vi "TLB Native Dynamic Events ver 0.05f.vi"() -> ()   [LabVIEW 2018]
uses:
  Labview Training Phase 2/Enum Controls/States for Action Engine.ctl
  Type def/TLB event states.ctl
  Type def/TLB MHL States.ctl
  <vilib>/Studica/Studica Toolkit/Background/I2C Channel.ctl
  <vilib>/Studica/Studica Toolkit/NavX/NavX.lvlib
  <vilib>/myRIO/Common/Instrument Driver Framework/myRIO v1.0/AI/typedefs/AI Channels Enum.ctl
  <vilib>/myRIO/Common/Instrument Driver Framework/myRIO v1.0/AI/typedefs/AI Channels List.ctl
  <vilib>/Studica/Studica Toolkit/Background/Mxp Selection.ctl
  <vilib>/ptbypt/NI_PtbyPt.lvlib
  Type def/Type def.ctl
  Type def/Motor Control Cluster.ctl
  <vilib>/Studica/Studica Blackhawk/Blackhawk.lvlib
  <vilib>/Studica/Studica Toolkit/Background/DIO Channel.ctl
panel:
  out "Image Processing error":errorcluster
  in  "Camera playback":bool
  out "Image Out":T1(plugin-control)
  out "element":T2
  in  "Servo Angle":u8(slide) scale=0.0..180.0
  in  "On/Off":bool
  out "Blackhawk error":errorcluster
  out "Value Read":bool
  out "Object detected":bool
  out "Yaw":dbl
  in  "NavX Zero Yaw":bool
  out "NavX Info Out":T4
  out "LinearAcceleration":T5
  out "Displacement":T6
  out "YRPHfH":T7
  out "Distance":T8
  in  "Return to IDLE":bool
  out "Right IR Sensor":dbl
  out "Left IR Sensor":dbl
  out "CM":fxp<+,64,16>
  out "Ultrasonic sensor":dbl format="%0.2f"
  in  "xTargetSpeed":dbl
  in  "yTargetSpeed":dbl
  in  "wTargetSpeed":dbl
  out "Speed":T9
  in  "Reset Encoder 0":bool
  out "Action Queue Items":i32
  out "State Logic Queue Items":i32
  out "Action Queues items":string[](array[string])=["Hardware reset", "Software reset", ""]
  out "State logic":T10=enum."Task 2"
  out "Action State":string
  in  "Tasks Selector":string(combo)="Task 2"
  in  "Stop Queue":bool
  in  "Start Task":bool
  # "Test Programme written by Calvin Loke    Dated: 28 Aug 2019\nTest Programme revised by Dr Alex See   Dated 30 Aug 2019\n\nProgramme version:   TLB Native Dynamic Events ver 0.04b.vi"
  # "Sequence of Actions"
  # "Continuous (Repeated)"
  # "System Health Status Update"
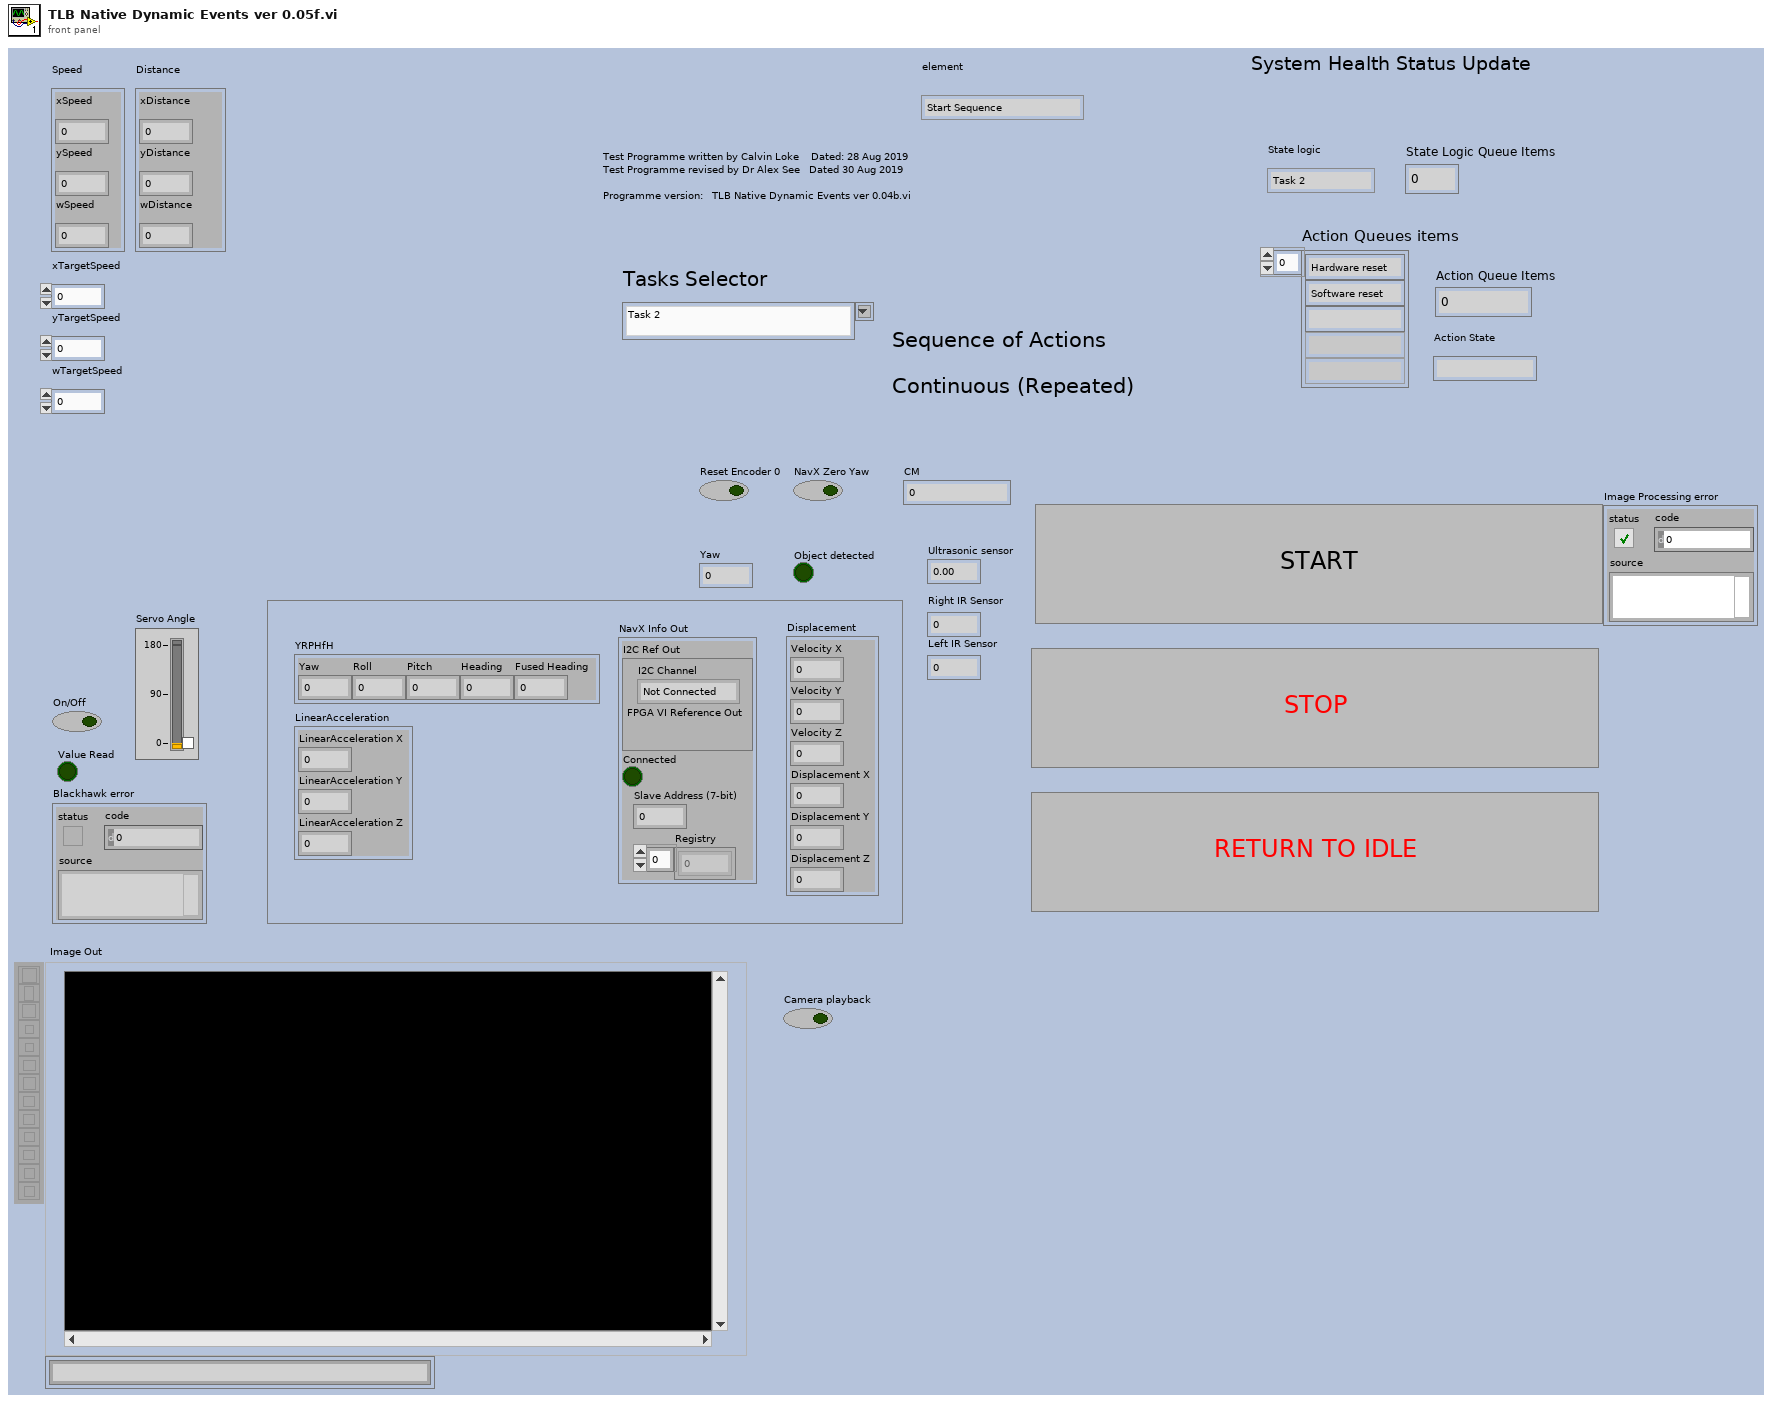
[diagram p1: front panel]
types:
  T1 = typedef "IMAQ Image.ctl" = refnum<image>
  T2 = typedef "TLB event states.ctl" = enum16{"Start Sequence", "Exit", "Start Task 1", "Start Task 2", "Start Task 3", "Start Task 4", "Camera vision", "Wall follow mode", "Idle", "Start Drive Straight"}
  T3 = typedef "I2C Channel.ctl" = enum16{"Not Connected", "A", "B"}
  T4 = cluster{"I2C Ref Out":cluster{"I2C Channel":T3, "FPGA VI Reference Out":refnum<k20>}, "Connected":bool, "Slave Address (7-bit)":u8, "Registry":u8[]}
  T5 = cluster{"LinearAcceleration X":dbl, "LinearAcceleration Y":dbl, "LinearAcceleration Z":dbl}
  T6 = cluster{"Velocity X":dbl, "Velocity Y":dbl, "Velocity Z":dbl, "Displacement X":dbl, "Displacement Y":dbl, "Displacement Z":dbl}
  T7 = cluster{"Yaw":dbl, "Roll":dbl, "Pitch":dbl, "Heading":dbl, "Fused Heading":dbl}
  T8 = cluster{"xDistance":dbl, "yDistance":dbl, "wDistance":dbl}
  T9 = cluster{"xSpeed":dbl, "ySpeed":dbl, "wSpeed":dbl}
  T10 = typedef "TLB MHL States.ctl" = enum16{"None", "Startup", "Idle", "Processing", "Shutdown", "Reset", "Task 1", "Task 2", "Task 3", "Task 4", "Task 4a", "Task 4b", "Task 4c", "Task 4d", "Task 4e", "Task 4f", "Task 4g", "Task 4h", "Acquire image", "Wall follow mode", "Autodrive", "Autodrive a"}
  T11 = typedef "States for Action Engine.ctl" = enum16{"Initialize", "Write", "Read"}
  T12 = typedef "DIO Channel.ctl" = enum16{"Not Connected", "A/DIO1", "A/DIO2", "A/DIO3", "A/DIO4", "A/DIO5", "A/DIO6", "A/DIO7", "A/DIO13", "B/DIO1", "B/DIO2", "B/DIO3", "B/DIO4", "B/DIO5", "B/DIO6", "B/DIO7", "B/DIO13", "C/DIO0", "C/DIO1", "C/DIO2", "C/DIO3", "C/DIO4", "C/DIO5", "C/DIO6", "C/DIO7"}
  T13 = typedef "Motor Control Cluster.ctl" = cluster{"Vx":dbl, "Vy":dbl, "Vw":dbl}
  T14 = typedef "Type def.ctl" = cluster{"Front Ultrasonic Obstruct":bool, "Left Ultrasonic Obstruct":bool, "Right Ultrasonic Obstruct ":bool}
  T15 = typedef "Mxp Selection.ctl" = enum16{"MXP A", "MXP B"}
  T16 = typedef "TLB event states.ctl" = enum16{"Start Sequence", "Exit", "Start Task 1", "Start Task 2", "Start Task 3", "Start Task 4", "RT Camera tracking", "Wall follow mode", "Idle"}
  T17 = cluster{"I2C Channel":T3, "FPGA VI Reference Out":refnum<k20>}
  T18 = typedef "AI Channels List.ctl" = T19[]
  T19 = typedef "AI Channels Enum.ctl" = enum16{"Not Connected", "AudioIn/Left", "AudioIn/Right", "C/AI0", "C/AI1", "A/AI0", "A/AI1", "A/AI2", "A/AI3", "A/AI4", "A/AI5", "A/AI6", "A/AI7", "B/AI0", "B/AI1", "B/AI2", "B/AI3", "B/AI4", "B/AI5", "B/AI6", "B/AI7", "AI/AI0", "AI/AI1", "AI/AI2", "AI/AI3", "A/AI0 (DIFF)", "A/AI1 (DIFF)", "A/AI2 (DIFF)", "A/AI3 (DIFF)", "B/AI0 (DIFF)", "B/AI1 (DIFF)", "B/AI2 (DIFF)", "B/AI3 (DIFF)"}
  T20 = cluster{"DIO Channel":T12, "FPGA VI Reference Out":refnum<k20>}
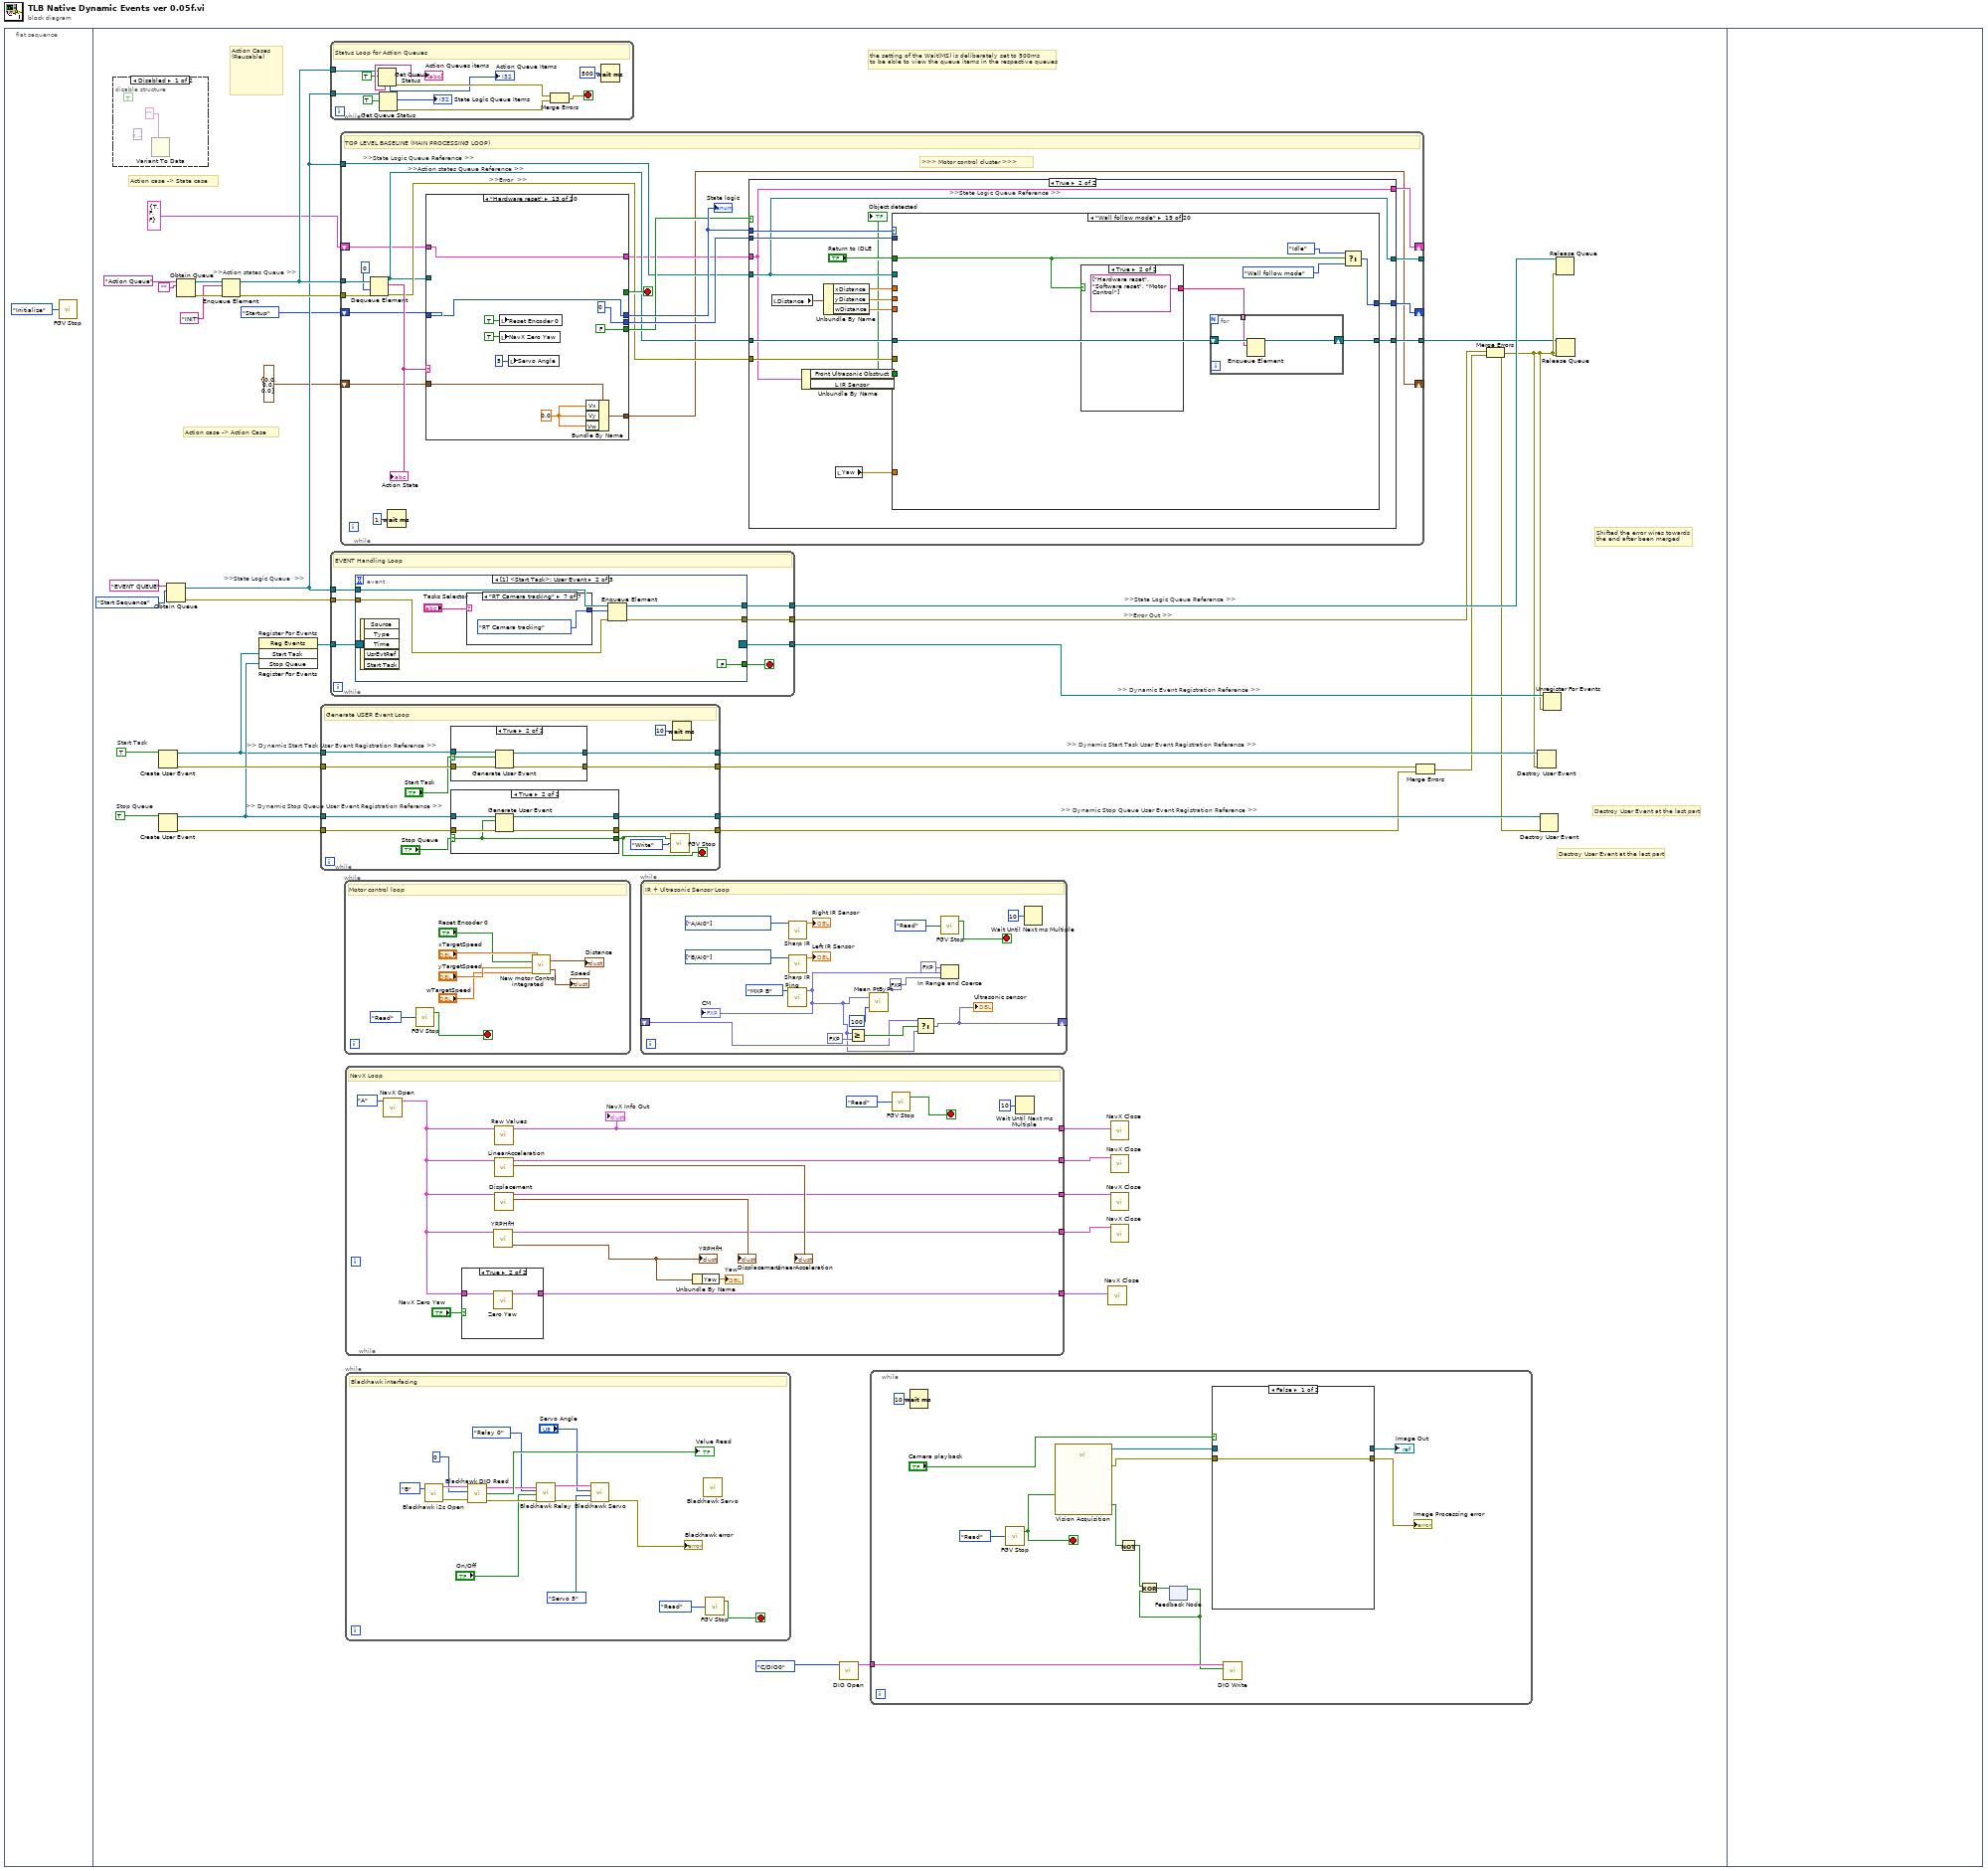
[diagram p0: block diagram]
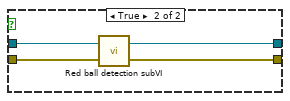
[diagram p2: hidden frame]
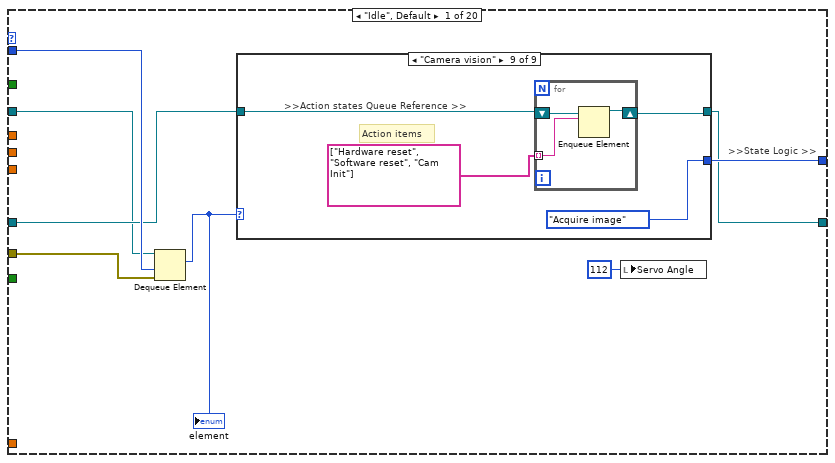
[diagram p6: hidden frame]
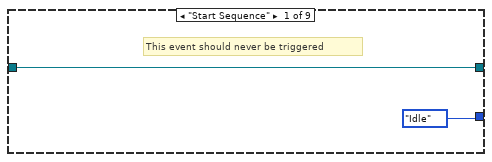
[diagram p7: hidden frame]
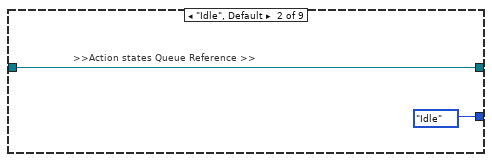
[diagram p8: hidden frame]
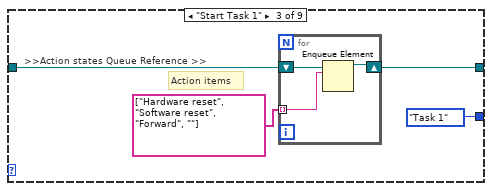
[diagram p9: hidden frame]
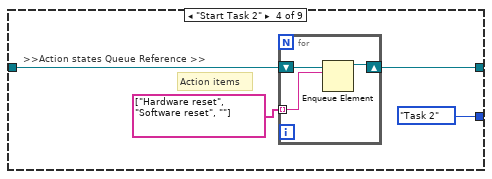
[diagram p10: hidden frame]
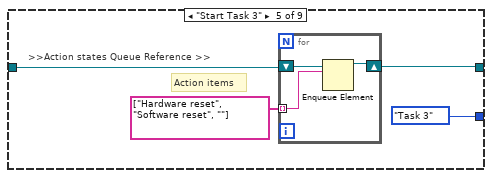
[diagram p11: hidden frame]
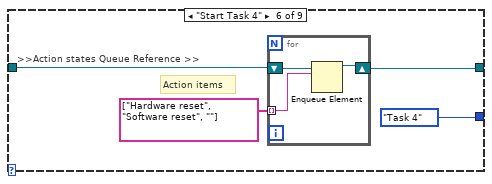
[diagram p12: hidden frame]
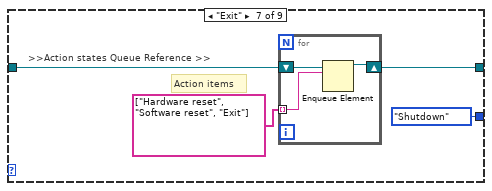
[diagram p13: hidden frame]
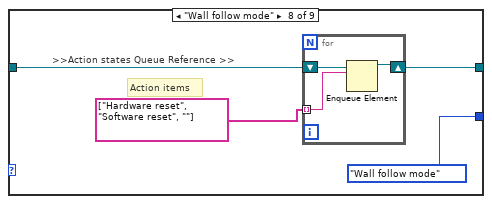
[diagram p14: hidden frame]
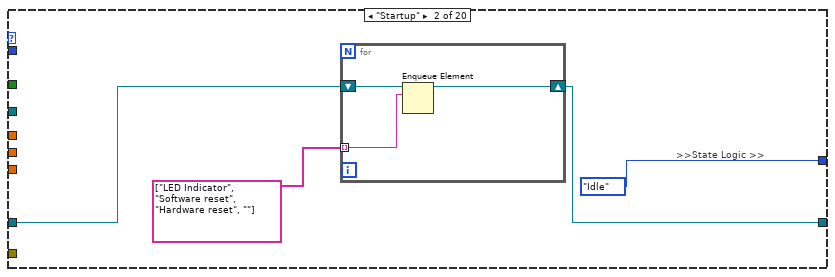
[diagram p15: hidden frame]
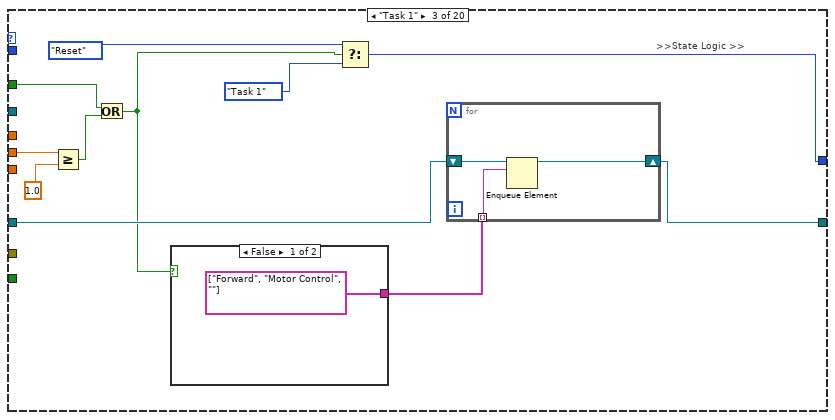
[diagram p16: hidden frame]
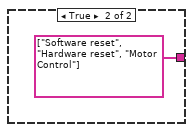
[diagram p17: hidden frame]
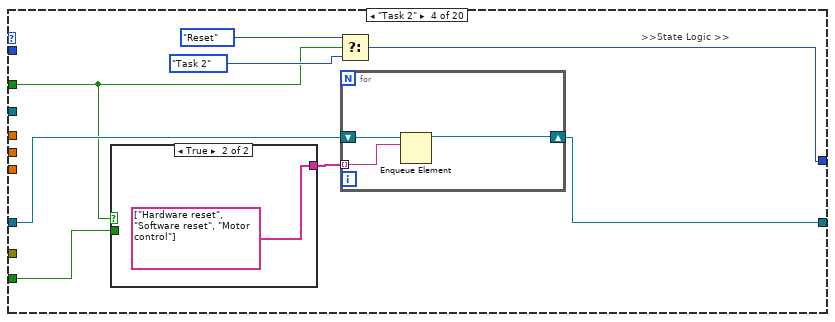
[diagram p18: hidden frame]
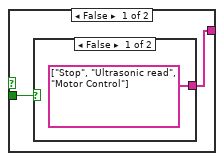
[diagram p19: hidden frame]
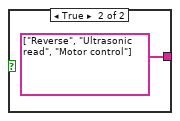
[diagram p20: hidden frame]
diagram:
  n1 = flat-sequence {
    frame #0 {
      n2 = call "FGV Stop.vi"("Init/Read/Write State"=States_for_Action_Engine."Initialize") -> ()  [unwired: 2 in, 2 out]
    }
    frame #1 {
      w39 = TRUE  # Stop Queue
      w38 = TRUE  # Start Task
      # "Action case -> Action Case"
      # "Action case -> State case"
      # "the setting of the Wait(MS) is deliberately set to 500ms\nto be able to view the queue items in the respective queues"
      # "Action Cases\n(Reusable)"
      # ">>Error Out >>"
      # ">> Dynamic Stop Queue User Event Registration Reference >>"
      # ">> Dynamic Start Task User Event Registration Reference >>"
      # ">> Dynamic Stop Queue User Event Registration Reference >>"
      # ">> Dynamic Start Task User Event Registration Reference >>"
      # ">> Dynamic Event Registration Reference >>"
      # ">>Action states Queue >>"
      # ">>State Logic Queue  >>"
      # ">>State Logic Queue Reference >>"
      # "Destroy User Event at the last part"
      # "Destroy User Event at the last part"
      # "Shifted the error wires towards\nthe end after been merged"
      n3 = disable-structure shown="Disabled" {
        frame Disabled {
          (unwired) variant
          (unwired) TRUE
          n4 = Variant To Data(type="") -> ()  [unwired: 2 in, 2 out]
        }
        frame Enabled {
        }
      }
      n5 = Create User Event(user event datatype=w38) -> (user event=w30:refnum<user-event>, error out=w35:errorcluster)  [unwired: 1 in]
      n6 = Create User Event(user event datatype=w39) -> (user event=w31:refnum<user-event>, error out=w34:errorcluster)  [unwired: 1 in]
      n7 = Obtain Queue(name (unnamed)="EVENT QUEUE", element data type=TLB_event_states."Start Sequence" ("Enum")) -> (queue out=w15:refnum<queue>, error out=w21:errorcluster)  [unwired: 3 in, 1 out]
      n8 = Obtain Queue(name (unnamed)="Action Queue", element data type="") -> (queue out=w24:refnum<queue>, error out=w20:errorcluster)  [unwired: 3 in, 1 out]
      n9 = Enqueue Element(queue=w24, element="INIT", error in (no error)=w20) -> (queue out=w16:refnum<queue>, error out=w19:errorcluster)  [unwired: 1 in, 1 out]
      n10 = register-events "Register For Events"(w30, w31) -> (reference out=w29:refnum<event-registration>)  [unwired: 2 in, 1 out]
      n11 = while {
        tunnel: w30 -> [w603]
        tunnel: w31 -> [w602]
        tunnel: [w601] -> w37
        tunnel: [w600] -> w36
        tunnel: w35 -> [w599]
        tunnel: [w598] -> w33
        tunnel: w34 -> [w597]
        tunnel: [w596] -> w32
        stop <- w592 stop-if-true
        # "Generate USER Event Loop"
        n12 = case shown="True" "Start Task" {
          selector: "Start Task" -> [_ w615]
          tunnel: w603 -> [w614 w619]
          tunnel: [w614 w618] -> w600
          tunnel: w599 -> [w613 w617]
          tunnel: [w613 w616] -> w598
          frame False {
          }
          frame True {
            n13 = Generate User Event(user event=w619, event data cluster=w615, error in=w617) -> (user event out=w618:refnum<user-event>, error out=w616:errorcluster)  [unwired: 1 in]
          }
        }
        n14 = case shown="True" "Stop Queue" {
          selector: "Stop Queue" -> [_ w608]
          tunnel: w602 -> [w607 w612]
          tunnel: [w607 w611] -> w601
          tunnel: w597 -> [w606 w610]
          tunnel: [w606 w609] -> w596
          tunnel: [FALSE w608] -> w592
          frame False {
          }
          frame True {
            n15 = Generate User Event(user event=w612, event data cluster=w608, error in=w610) -> (user event out=w611:refnum<user-event>, error out=w609:errorcluster)  [unwired: 1 in]
          }
        }
        n16 = call "FGV Stop.vi"("Init/Read/Write State"=States_for_Action_Engine."Write", "Input Node"=w592) -> ()  [unwired: 1 in, 2 out]
        n17 = Wait (ms)(milliseconds to wait=u32 10) -> ()  [unwired: 1 out]
      }
      n18 = while {
        tunnel: w16 -> [w125]
        tunnel: w15 -> [w122]
        stop <- w119 stop-if-true
        # "Status Loop for Action Queues"
        n19 = Get Queue Status(queue=w125, return elements? (F)=TRUE) -> (error out=w121:errorcluster, # elements in queue=→"Action Queue Items":i32, elements=→"Action Queues items":string[])  [unwired: 1 in, 5 out]
        n20 = Get Queue Status(queue=w122, return elements? (F)=TRUE) -> (# pending remove=→"State Logic Queue Items":i32, error out=w120:errorcluster)  [unwired: 1 in, 6 out]
        n21 = Merge Errors(w121, w120) -> (w119:errorcluster)
        n22 = Wait (ms)(milliseconds to wait=u32 500) -> ()  [unwired: 1 out]
      }
      n23 = while {
        tunnel: w29 -> [w565]
        tunnel: [w564] -> w28
        tunnel: w15 -> [w562]
        tunnel: [w561] -> w27
        tunnel: w21 -> [w560]
        tunnel: [w559] -> w18
        stop <- w563 stop-if-true
        # "EVENT Handling Loop"
        n24 = event shown="[1] <Start Task>: User Event" {
          selector: w565 -> [_ _ _]
          dyn-events: [_ _ _] -> w564
          timeout: _ -> [_ _ _]
          tunnel: [FALSE FALSE w591] -> w563
          tunnel: w562 -> [w570 w577 w589]
          tunnel: [w569 w576 w590] -> w561
          tunnel: w560 -> [w567 w573 w587]
          tunnel: [w566 w572 w586] -> w559
          event Timeout {
            n25 = event-data() -> ()  [unwired: 1 in, 3 out]
            n26 = Enqueue Element(queue=w570, element=TLB_event_states."Idle" ("Enum"), error in (no error)=w567) -> (queue out=w569:refnum<queue>, error out=w566:errorcluster)  [unwired: 1 in, 1 out]
          }
          event User Event {
            n27 = event-data() -> ()  [unwired: 1 in, 5 out]
            n28 = case shown="\"RT Camera tracking\"" "Tasks Selector" {
              tunnel: [TLB_event_states."Idle" ("Enum") TLB_event_states."Start Task 1" ("Enum") TLB_event_states."Start Task 2" ("Enum") TLB_event_states."Start Task 3" ("Enum") TLB_event_states."Start Task 4" ("Enum") TLB_event_states."Wall follow mode" ("Enum") TLB_event_states."RT Camera tracking" ("Enum")] -> w574
              frame Default {
              }
              frame "Task 1" {
              }
              frame "Task 2" {
              }
              frame "Task 3" {
              }
              frame "Task 4" {
              }
              frame "Wall following" {
              }
              frame "RT Camera tracking" {
              }
            }
            n29 = Enqueue Element(queue=w577, element=w574, error in (no error)=w573) -> (queue out=w576:refnum<queue>, error out=w572:errorcluster)  [unwired: 1 in, 1 out]
          }
          event User Event {
            n30 = event-data() -> ("Stop Queue"=w591:bool)  [unwired: 1 in, 4 out]
            n31 = Enqueue Element At Opposite End(queue=w589, element=TLB_event_states."Exit" ("Enum"), error in (no error)=w587) -> (queue out=w590:refnum<queue>, error out=w586:errorcluster)  [unwired: 1 in, 1 out]
          }
        }
      }
      n32 = while {
        tunnel: w15 -> [w136]
        shift-right: [w141] -> _
        shift-left: TLB_MHL_States."Startup" ("Enum") -> [w133]
        tunnel: w16 -> [w146]
        tunnel: w19 -> [w144]
        tunnel: [w143] -> _
        tunnel: [w142] -> w13
        shift-right: [w130] -> _
        shift-left: T14 {"Front Ultrasonic Obstruct"=TRUE, "Left Ultrasonic Obstruct"=FALSE, "Right Ultrasonic Obstruct "=FALSE} -> [w132]
        shift-right: [w128] -> _
        shift-left: T13 {"Vx"=0.0, "Vy"=0.0, "Vw"=0.0} -> [w129]
        stop <- w139 stop-if-true
        # ">>> Motor control cluster >>>"
        # ">>Error  >>"
        # ">>Action states Queue Reference >>"
        # ">>State Logic Queue Reference >>"
        # "TOP LEVEL BASELINE (MAIN PROCESSING LOOP)"
        n33 = Dequeue Element(queue=w146, timeout in ms (-1)=0, error in (no error)=w144) -> (queue out=w134:refnum<queue>, element=w145:string, error out=w135:errorcluster)  [unwired: 1 out]
        "Action State" <- w145
        n34 = Wait (ms)(milliseconds to wait=u32 1) -> ()  [unwired: 1 out]
        n35 = case shown="\"Hardware reset\"" w145 {
          tunnel: [w405 w412 w417 w425 w434 w444 w453 w460 w471 w479 w487 w496 w506 TLB_MHL_States."Shutdown" ("Enum") w521 w525 w539 w545 w549 w558] -> w147
          tunnel: [w404 0 0 0 0 0 0 0 0 0 0 0 0 0 0 0 0 0 0 0] -> w140
          tunnel: [_ _ _ _ _ _ _ _ _ _ _ _ _ TRUE _ _ _ _ _ _] -> w139
          tunnel: [TRUE FALSE FALSE FALSE FALSE FALSE FALSE FALSE FALSE FALSE FALSE FALSE FALSE FALSE FALSE FALSE FALSE FALSE FALSE FALSE] -> w138
          tunnel: w134 -> [_ _ _ _ _ _ _ _ _ _ _ _ _ _ _ _ _ _ _ _]
          tunnel: w133 -> [w405 w412 w417 w425 w434 w444 w453 w460 w471 w479 w487 w496 w506 _ w521 w525 w539 w545 w549 w558]
          tunnel: w132 -> [w402 w409 w414 w421 w430 w439 w448 w457 w466 w475 w488 w493 w501 w508 w520 w528 w540 w546 w547 w553]
          tunnel: [w402 w409 w414 w421 w430 w439 w448 w457 w466 w475 w488 w492 w501 w508 w517 w527 w540 w546 w547 w553] -> w131
          tunnel: w129 -> [w401 w408 w413 w419 w428 w437 w447 w455 w465 w473 w481 w490 w500 w507 w513 w522 w531 w544 w552 w555]
          tunnel: [w401 w408 w413 w420 w429 w438 w446 w456 w464 w474 w481 w490 w498 w507 w513 w522 w532 w544 w552 w555] -> w128
          frame "No action", Default {
            n36 = case shown="\"Startup\", Default" w405 {
              tunnel: [0 100] -> w404
              frame "Startup", Default {
              }
              frame "Idle" {
              }
            }
          }
          frame "Init" {
            # ">>State Logic  >>"
          }
          frame "LED Indicator" {
          }
          frame "Forward" {
            n37 = local write "Reset Encoder 0"(FALSE ("Reset Encoder 0")) -> ()
            n38 = local write "NavX Zero Yaw"(FALSE ("NavX Zero Yaw")) -> ()
            n39 = Bundle By Name(cluster=w419, "Vy"=0.6) -> (w420:T13)
          }
          frame "Reverse" {
            n40 = local write "NavX Zero Yaw"(FALSE ("NavX Zero Yaw")) -> ()
            n41 = local write "Reset Encoder 0"(FALSE ("Reset Encoder 0")) -> ()
            n42 = Bundle By Name(cluster=w428, "Vy"=-0.6) -> (w429:T13)
          }
          frame "Right" {
            n43 = local write "NavX Zero Yaw"(FALSE ("NavX Zero Yaw")) -> ()
            n44 = local write "Reset Encoder 0"(FALSE ("Reset Encoder 0")) -> ()
            n45 = Bundle By Name(cluster=w437, "Vx"=0.6) -> (w438:T13)
          }
          frame "Left" {
            n46 = Bundle By Name(cluster=w447, "Vx"=-0.6) -> (w446:T13)
            n47 = local write "NavX Zero Yaw"(FALSE ("NavX Zero Yaw")) -> ()
            n48 = local write "Reset Encoder 0"(FALSE ("Reset Encoder 0")) -> ()
          }
          frame "Rotate CW" {
            n49 = local write "NavX Zero Yaw"(FALSE ("NavX Zero Yaw")) -> ()
            n50 = local write "Reset Encoder 0"(FALSE ("Reset Encoder 0")) -> ()
            n51 = Bundle By Name(cluster=w455, "Vw"=-0.3) -> (w456:T13)
          }
          frame "Rotate ACW" {
            n52 = local write "Reset Encoder 0"(FALSE ("Reset Encoder 0")) -> ()
            n53 = local write "NavX Zero Yaw"(FALSE ("NavX Zero Yaw")) -> ()
            n54 = Bundle By Name(cluster=w465, "Vw"=0.15) -> (w464:T13)
          }
          frame "Stop" {
            w472 = 0.0
            n55 = local write "NavX Zero Yaw"(FALSE ("NavX Zero Yaw")) -> ()
            n56 = local write "Reset Encoder 0"(FALSE ("Reset Encoder 0")) -> ()
            n57 = Bundle By Name(cluster=w473, "Vx"=w472, "Vy"=w472, "Vw"=w472) -> (w474:T13)
          }
          frame "Motor control" {
            # "Replace with FGV"
            n58 = Unbundle By Name(w481) -> ("Vx"=w484:dbl, "Vy"=w483:dbl, "Vw"=w482:dbl)
            n59 = local write "xTargetSpeed"(w484) -> ()
            n60 = local write "yTargetSpeed"(w483) -> ()
            n61 = local write "wTargetSpeed"(w482) -> ()
          }
          frame "Software reset" {
            w491 = FALSE ("NavX Zero Yaw")
            n62 = local write "NavX Zero Yaw"(w491) -> ()
            n63 = Bundle By Name(cluster=w493, "Front Ultrasonic Obstruct"=w491, "L IR Sensor"=0.0) -> (w492:T14)
          }
          frame "Hardware reset" {
            w499 = 0.0
            n64 = local write "Reset Encoder 0"(TRUE ("Reset Encoder 0")) -> ()
            n65 = local write "NavX Zero Yaw"(TRUE ("NavX Zero Yaw")) -> ()
            n66 = local write "Servo Angle"(u8 5 ("Servo Angle")) -> ()
            n67 = Bundle By Name(cluster=w500, "Vx"=w499, "Vy"=w499, "Vw"=w499) -> (w498:T13)
          }
          frame "Exit" {
          }
          frame "Ultrasonic read" {
            # "Object detection"
            n68 = local read "Ultrasonic sensor"() -> (w516:dbl)
            n69 = Less Or Equal?(x=w516, y=20.0) -> (x <= y?=w514:bool)
            n70 = Bundle By Name(cluster=w520, "Front Ultrasonic Obstruct"=w514) -> (w517:T14)
          }
          frame "IR Sensor Read" {
            n71 = local read "Left IR Sensor"() -> (w526:dbl)
            n72 = Bundle By Name(cluster=w528, "L IR Sensor"=w526) -> (w527:T14)
          }
          frame "Calculate" {
            n73 = Unbundle By Name(w540) -> ("L IR Sensor"=w536:dbl)
            n74 = Subtract(x=w536, y=20.0) -> (x-y=w534:dbl)
            n75 = Multiply(x=w534, y=0.01) -> (x*y=w530:dbl)
            n76 = Bundle By Name(cluster=w531, "Vy"=0.4, "Vw"=w530) -> (w532:T13)
          }
          frame "Cam Init" {
            n77 = local write "Camera playback"(TRUE ("Camera playback")) -> ()
          }
          frame "Cam Acq" {
            n78 = local write "Camera playback"(TRUE ("Camera playback")) -> ()
          }
          frame "Cam Exit" {
            n79 = local write "Camera playback"(FALSE ("Camera playback")) -> ()
          }
        }
        "State logic" <- w147
        n80 = case shown="True" w138 {
          tunnel: w147 -> [w151 w167]
          tunnel: w136 -> [w152 w161]
          tunnel: w134 -> [w150 w166]
          tunnel: [w152 w161] -> w143
          tunnel: [w150 w165] -> w142
          tunnel: [w151 w164] -> w141
          tunnel: w135 -> [_ w163]
          tunnel: w140 -> [_ w162]
          tunnel: w131 -> [w149 w153]
          tunnel: [w149 w153] -> w130
          frame False {
          }
          frame True {
            # ">>State Logic Queue Reference >>"
            n81 = local read "Distance"() -> (w159:T8)
            n82 = Unbundle By Name(w153) -> ("Front Ultrasonic Obstruct"=w154:bool)  [unwired: 1 out]
            "Object detected" <- w154
            n83 = Unbundle By Name(w159) -> ("xDistance"=w156:dbl, "yDistance"=w158:dbl, "wDistance"=w157:dbl)
            n84 = local read "Yaw"() -> (w155:dbl)
            n85 = case shown="\"Wall follow mode\"" w167 {
              tunnel: w161 -> [w169 _ _ _ _ _ _ _ _ _ _ _ _ _ _ _ _ _ _ _]
              tunnel: w166 -> [w171 w230 w242 w255 w277 w286 w300 w315 w328 w341 w352 w358 w361 w367 w370 w372 w374 w376 w379 w393]
              tunnel: [w170 w229 w241 w256 w276 w287 w299 w314 w327 w340 w351 w358 w360 w367 w370 w372 w374 w376 w380 w392] -> w165
              tunnel: [w174 TLB_MHL_States."Idle" ("Enum") w244 w257 w273 w290 w302 w313 w329 w339 TLB_MHL_States."Idle" ("Enum") TLB_MHL_States."Reset" ("Enum") TLB_MHL_States."Shutdown" ("Enum") TLB_MHL_States."Reset" ("Enum") TLB_MHL_States."Idle" ("Enum") TLB_MHL_States."Idle" ("Enum") TLB_MHL_States."Idle" ("Enum") TLB_MHL_States."Idle" ("Enum") w382 w391] -> w164
              tunnel: w163 -> [w172 _ _ _ _ _ _ _ _ _ _ _ _ _ _ _ _ _ _ _]
              tunnel: w162 -> [w173 _ _ _ _ _ _ _ _ _ _ _ _ _ _ _ _ _ _ _]
              tunnel: "Return to IDLE" -> [_ _ w239 w254 w271 _ _ _ _ _ _ _ _ _ _ _ _ _ w377 w390]
              tunnel: w158 -> [_ _ w238 _ _ _ _ w312 _ _ _ _ _ _ _ _ _ _ _ _]
              tunnel: w157 -> [_ _ _ _ w270 _ _ _ _ _ _ _ _ _ _ _ _ _ _ _]
              tunnel: w156 -> [_ _ _ _ _ _ w296 _ w324 _ _ _ _ _ _ _ _ _ _ _]
              tunnel: w155 -> [_ _ _ _ _ _ _ _ _ _ _ _ _ _ _ _ _ _ _ _]
              tunnel: w154 -> [_ _ _ w252 _ w284 _ _ _ w338 _ _ _ _ _ _ _ _ _ _]
              frame "Idle", Default {
                # ">>State Logic >>"
                n86 = Dequeue Element(queue=w169, timeout in ms (-1)=w173, error in (no error)=w172) -> (element=w175:T2)  [unwired: 3 out]
                "element" <- w175
                n87 = case shown="\"Camera vision\"" w175 {
                  tunnel: [TLB_MHL_States."Idle" ("Enum") TLB_MHL_States."Idle" ("Enum") TLB_MHL_States."Task 1" ("Enum") TLB_MHL_States."Task 2" ("Enum") TLB_MHL_States."Task 3" ("Enum") TLB_MHL_States."Task 4" ("Enum") TLB_MHL_States."Shutdown" ("Enum") TLB_MHL_States."Wall follow mode" ("Enum") TLB_MHL_States."Acquire image" ("Enum")] -> w174
                  tunnel: [w177 w178 w182 w187 w196 w202 w208 w215 w223] -> w170
                  tunnel: w171 -> [w177 w178 w180 w188 w197 w203 w209 w216 w224]
                  frame "Start Sequence" {
                    # "This event should never be triggered"
                  }
                  frame "Idle", Default {
                    # ">>Action states Queue Reference >>"
                  }
                  frame "Start Task 1" {
                    # ">>Action states Queue Reference >>"
                    # "Action items"
                    n88 = for {
                      shift-right: [w186] -> w182
                      shift-left: w180 -> [w185]
                      tunnel: string[] ["Hardware reset", "Software reset", "Forward", ""] -> [w184] mode=indexing
                      n89 = Enqueue Element(queue=w185, element=w184) -> (queue out=w186:refnum<queue>)  [unwired: 2 in, 2 out]
                    }
                  }
                  frame "Start Task 2" {
                    # ">>Action states Queue Reference >>"
                    # "Action items"
                    n90 = for {
                      shift-right: [w193] -> w187
                      shift-left: w188 -> [w192]
                      tunnel: string[] ["Hardware reset", "Software reset", ""] -> [w191] mode=indexing
                      n91 = Enqueue Element(queue=w192, element=w191) -> (queue out=w193:refnum<queue>)  [unwired: 2 in, 2 out]
                    }
                  }
                  frame "Start Task 3" {
                    # ">>Action states Queue Reference >>"
                    # "Action items"
                    n92 = for {
                      shift-right: [w200] -> w196
                      shift-left: w197 -> [w199]
                      tunnel: string[] ["Hardware reset", "Software reset", ""] -> [w198] mode=indexing
                      n93 = Enqueue Element(queue=w199, element=w198) -> (queue out=w200:refnum<queue>)  [unwired: 2 in, 2 out]
                    }
                  }
                  frame "Start Task 4" {
                    # ">>Action states Queue Reference >>"
                    # "Action items"
                    n94 = for {
                      shift-right: [w207] -> w202
                      shift-left: w203 -> [w206]
                      tunnel: string[] ["Hardware reset", "Software reset", ""] -> [w205] mode=indexing
                      n95 = Enqueue Element(queue=w206, element=w205) -> (queue out=w207:refnum<queue>)  [unwired: 2 in, 2 out]
                    }
                  }
                  frame "Exit" {
                    # ">>Action states Queue Reference >>"
                    # "Action items"
                    n96 = for {
                      shift-right: [w214] -> w208
                      shift-left: w209 -> [w213]
                      tunnel: string[] ["Hardware reset", "Software reset", "Exit"] -> [w212] mode=indexing
                      n97 = Enqueue Element(queue=w213, element=w212) -> (queue out=w214:refnum<queue>)  [unwired: 2 in, 2 out]
                    }
                  }
                  frame "Wall follow mode" {
                    # ">>Action states Queue Reference >>"
                    # "Action items"
                    n98 = for {
                      shift-right: [w221] -> w215
                      shift-left: w216 -> [w220]
                      tunnel: string[] ["Hardware reset", "Software reset", ""] -> [w219] mode=indexing
                      n99 = Enqueue Element(queue=w220, element=w219) -> (queue out=w221:refnum<queue>)  [unwired: 2 in, 2 out]
                    }
                  }
                  frame "Camera vision" {
                    # ">>Action states Queue Reference >>"
                    # "Action items"
                    n100 = for {
                      shift-right: [w228] -> w223
                      shift-left: w224 -> [w227]
                      tunnel: string[] ["Hardware reset", "Software reset", "Cam Init"] -> [w226] mode=indexing
                      n101 = Enqueue Element(queue=w227, element=w226) -> (queue out=w228:refnum<queue>)  [unwired: 2 in, 2 out]
                    }
                  }
                }
                n102 = local write "Servo Angle"(u8 112 ("Servo Angle")) -> ()
              }
              frame "Startup" {
                # ">>State Logic >>"
                n103 = for {
                  shift-right: [w234] -> w229
                  shift-left: w230 -> [w235]
                  tunnel: string[] ["LED Indicator", "Software reset", "Hardware reset", ""] -> [w233] mode=indexing
                  n104 = Enqueue Element(queue=w235, element=w233) -> (queue out=w234:refnum<queue>)  [unwired: 2 in, 2 out]
                }
              }
              frame "Task 1" {
                # ">>State Logic >>"
                n105 = Greater Or Equal?(x=w238, y=1.0) -> (x >= y?=w236:bool)
                n106 = Or(x=w239, y=w236) -> (x .or. y?=w240:bool)
                n107 = case shown="False" w240 {
                  tunnel: [string[] ["Forward", "Motor Control", ""] string[] ["Software reset", "Hardware reset", "Motor Control"]] -> w243
                  frame False {
                  }
                  frame True {
                  }
                }
                n108 = Select(t=TLB_MHL_States."Reset" ("Enum"), s=w240, f=TLB_MHL_States."Task 1" ("Enum")) -> (s? t:f=w244:T10)
                n109 = for {
                  shift-right: [w250] -> w241
                  shift-left: w242 -> [w251]
                  tunnel: w243 -> [w249] mode=indexing
                  n110 = Enqueue Element(queue=w251, element=w249) -> (queue out=w250:refnum<queue>)  [unwired: 2 in, 2 out]
                }
              }
              frame "Task 2" {
                # ">>State Logic >>"
                n111 = case shown="True" w254 {
                  tunnel: [w261 string[] ["Hardware reset", "Software reset", "Motor control"]] -> w253
                  tunnel: w252 -> [w260 _]
                  frame False {
                    n112 = case shown="False" w260 {
                      tunnel: [string[] ["Stop", "Ultrasonic read", "Motor Control"] string[] ["Reverse", "Ultrasonic read", "Motor control"]] -> w261
                      frame False {
                      }
                      frame True {
                      }
                    }
                  }
                  frame True {
                  }
                }
                n113 = Select(t=TLB_MHL_States."Reset" ("Enum"), s=w254, f=TLB_MHL_States."Task 2" ("Enum")) -> (s? t:f=w257:T10)
                n114 = for {
                  shift-right: [w266] -> w256
                  shift-left: w255 -> [w267]
                  tunnel: w253 -> [w265] mode=indexing
                  n115 = Enqueue Element(queue=w267, element=w265) -> (queue out=w266:refnum<queue>)  [unwired: 2 in, 2 out]
                }
              }
              frame "Task 3" {
                n116 = Less Or Equal?(x=w270, y=-1.2) -> (x <= y?=w268:bool)
                n117 = Or(x=w268, y=w271) -> (x .or. y?=w272:bool)
                n118 = case shown="True" w272 {
                  tunnel: [string[] ["Rotate CW", "Motor Control"] string[] ["Software reset", "Hardware reset", "Motor Control"]] -> w278
                  frame False {
                  }
                  frame True {
                  }
                }
                n119 = for {
                  shift-right: [w280] -> w276
                  shift-left: w277 -> [w281]
                  tunnel: w278 -> [w279] mode=indexing
                  n120 = Enqueue Element(queue=w281, element=w279) -> (queue out=w280:refnum<queue>)  [unwired: 2 in, 2 out]
                }
                n121 = Select(t=TLB_MHL_States."Reset" ("Enum"), s=w272, f=TLB_MHL_States."Task 3" ("Enum")) -> (s? t:f=w273:T10)
              }
              frame "Task 4" {
                n122 = case shown="False" w284 {
                  tunnel: [string[] ["Forward", "Ultrasonic read", "Motor Control"] string[] ["Stop", "Hardware reset", "Software reset", "Motor Control"]] -> w285
                  frame False {
                  }
                  frame True {
                  }
                }
                n123 = for {
                  shift-right: [w294] -> w287
                  shift-left: w286 -> [w295]
                  tunnel: w285 -> [w293] mode=indexing
                  n124 = Enqueue Element(queue=w295, element=w293) -> (queue out=w294:refnum<queue>)  [unwired: 2 in, 2 out]
                }
                n125 = Select(t=TLB_MHL_States."Task 4a" ("Enum"), s=w284, f=TLB_MHL_States."Task 4" ("Enum")) -> (s? t:f=w290:T10)
              }
              frame "Task 4a" {
                n126 = Greater Or Equal?(x=w296, y=0.5) -> (x >= y?=w298:bool)
                n127 = case shown="True" w298 {
                  tunnel: [string[] ["Right", "Motor Control"] string[] ["Stop", "Hardware reset", "Software reset", "Motor Control"]] -> w301
                  frame False {
                  }
                  frame True {
                  }
                }
                n128 = for {
                  shift-right: [w308] -> w299
                  shift-left: w300 -> [w309]
                  tunnel: w301 -> [w307] mode=indexing
                  n129 = Enqueue Element(queue=w309, element=w307) -> (queue out=w308:refnum<queue>)  [unwired: 2 in, 2 out]
                }
                n130 = Select(t=TLB_MHL_States."Task 4b" ("Enum"), s=w298, f=TLB_MHL_States."Task 4a" ("Enum")) -> (s? t:f=w302:T10)
              }
              frame "Task 4b" {
                n131 = Greater Or Equal?(x=w312, y=0.75) -> (x >= y?=w310:bool)
                n132 = case shown="False" w310 {
                  tunnel: [string[] ["Forward"] string[] ["Stop", "Hardware reset", "Software reset"]] -> w316
                  frame False {
                  }
                  frame True {
                  }
                }
                n133 = for {
                  shift-right: [w322] -> w314
                  shift-left: w315 -> [w323]
                  tunnel: w316 -> [w321] mode=indexing
                  n134 = Enqueue Element(queue=w323, element=w321) -> (queue out=w322:refnum<queue>)  [unwired: 2 in, 2 out]
                }
                n135 = Select(t=TLB_MHL_States."Task 4c" ("Enum"), s=w310, f=TLB_MHL_States."Task 4b" ("Enum")) -> (s? t:f=w313:T10)
              }
              frame "Task 4c" {
                n136 = Less Or Equal?(x=w324, y=-0.65) -> (x <= y?=w325:bool)
                n137 = case shown="False" w325 {
                  tunnel: [string[] ["Left"] string[] ["Stop", "Hardware reset", "Software reset"]] -> w330
                  frame False {
                  }
                  frame True {
                  }
                }
                n138 = for {
                  shift-right: [w336] -> w327
                  shift-left: w328 -> [w337]
                  tunnel: w330 -> [w335] mode=indexing
                  n139 = Enqueue Element(queue=w337, element=w335) -> (queue out=w336:refnum<queue>)  [unwired: 2 in, 2 out]
                }
                n140 = Select(t=TLB_MHL_States."Task 4d" ("Enum"), s=w325, f=TLB_MHL_States."Task 4c" ("Enum")) -> (s? t:f=w329:T10)
              }
              frame "Task 4d" {
                n141 = case shown="False" w338 {
                  tunnel: [string[] ["Forward", "Ultrasonic Read"] string[] ["Stop", "Hardware reset", "Software reset"]] -> w342
                  frame False {
                  }
                  frame True {
                  }
                }
                n142 = for {
                  shift-right: [w348] -> w340
                  shift-left: w341 -> [w349]
                  tunnel: w342 -> [w347] mode=indexing
                  n143 = Enqueue Element(queue=w349, element=w347) -> (queue out=w348:refnum<queue>)  [unwired: 2 in, 2 out]
                }
                n144 = Select(t=TLB_MHL_States."Task 4e" ("Enum"), s=w338, f=TLB_MHL_States."Task 4d" ("Enum")) -> (s? t:f=w339:T10)
              }
              frame "Reset" {
                n145 = for {
                  shift-right: [w356] -> w351
                  shift-left: w352 -> [w357]
                  tunnel: string[] ["Software reset", "Hardware reset", ""] -> [w355] mode=indexing
                  n146 = Enqueue Element(queue=w357, element=w355) -> (queue out=w356:refnum<queue>)  [unwired: 2 in, 2 out]
                }
                n147 = Wait (ms)(milliseconds to wait=u32 250) -> ()  [unwired: 1 out]
              }
              frame "Processing" {
              }
              frame "Shutdown" {
                # ">>State Logic >>"
                n148 = for {
                  shift-right: [w365] -> w360
                  shift-left: w361 -> [w366]
                  tunnel: string[] ["Software reset", "Hardware reset", "Cam Exit", "Exit"] -> [w364] mode=indexing
                  n149 = Enqueue Element(queue=w366, element=w364) -> (queue out=w365:refnum<queue>)  [unwired: 2 in, 2 out]
                }
              }
              frame "None" {
              }
              frame "Task 4e" {
              }
              frame "Task 4f" {
              }
              frame "Task 4g" {
              }
              frame "Task 4h" {
              }
              frame "Wall follow mode" {
                n150 = case shown="True" w377 {
                  tunnel: [string[] ["IR Sensor Read", "Calculate", "Forward", "Motor Control"] string[] ["Hardware reset", "Software reset", "Motor Control"]] -> w378
                  frame False {
                  }
                  frame True {
                  }
                }
                n151 = for {
                  shift-right: [w387] -> w380
                  shift-left: w379 -> [w388]
                  tunnel: w378 -> [w386] mode=indexing
                  n152 = Enqueue Element(queue=w388, element=w386) -> (queue out=w387:refnum<queue>)  [unwired: 2 in, 2 out]
                }
                n153 = Select(t=TLB_MHL_States."Idle" ("Enum"), s=w377, f=TLB_MHL_States."Wall follow mode" ("Enum")) -> (s? t:f=w382:T10)
              }
              frame "Acquire image" {
                n154 = case shown="False" w390 {
                  tunnel: [_ string[] ["Hardware reset", "Software reset", "Cam Exit", ""]] -> w394
                  frame False {
                  }
                  frame True {
                  }
                }
                n155 = for {
                  shift-right: [w399] -> w392
                  shift-left: w393 -> [w400]
                  tunnel: w394 -> [w398] mode=indexing
                  n156 = Enqueue Element(queue=w400, element=w398) -> (queue out=w399:refnum<queue>)  [unwired: 2 in, 2 out]
                }
                n157 = local write "Servo Angle"(u8 5 ("Servo Angle")) -> ()
                n158 = Select(t=TLB_MHL_States."Idle" ("Enum"), s=w390, f=TLB_MHL_States."Acquire image" ("Enum")) -> (s? t:f=w391:T10)
              }
            }
          }
        }
      }
      n159 = while {
        stop <- w115 stop-if-true
        # "Motor control loop"
        n160 = call "FGV Stop.vi"("Init/Read/Write State"=States_for_Action_Engine."Read") -> ("Output node"=w115:bool)  [unwired: 2 in, 1 out]
        n161 = call "New motor Control integrated.vi"("wTargetSpeed"="wTargetSpeed", "yTargetSpeed"="yTargetSpeed", "xTargetSpeed"="Reset Encoder 0", "Reset Encoders"="xTargetSpeed") -> ("Speed"=→"Speed":T9, "Distance"=→"Distance":T8)
      }
      n162 = while {
        tunnel: [w85] -> w9
        tunnel: [w82] -> w8
        tunnel: [w81] -> w6
        tunnel: [w80] -> w7
        tunnel: [w77] -> w5
        stop <- w87 stop-if-true
        # "NavX Loop"
        n163 = call <vilib>:"NavX Open.vi"("I2C Channel"=I2C_Channel."A") -> ("NavX Info"=w78:T4)  [unwired: 9 in, 1 out]
        n164 = case shown="True" "NavX Zero Yaw" {
          tunnel: w78 -> [w89 w91]
          tunnel: [w89 w90] -> w77
          frame False {
          }
          frame True {
            n165 = call <vilib>:"Zero Yaw.vi"("NavX Info In"=w91) -> ("NavX Info Out"=w90:T4)  [unwired: 10 in]
          }
        }
        n166 = call <vilib>:"YRPHfH.vi"("NavX Info In"=w78) -> ("YRPHfH"=w75:T7, "NavX Info Out"=w81:T4)  [unwired: 3 in]
        "YRPHfH" <- w75
        n167 = call <vilib>:"Raw Values.vi"("NavX Info In"=w78) -> ("NavX Info Out"=w85:T4)  [unwired: 8 in, 1 out]
        "NavX Info Out" <- w85
        n168 = call <vilib>:"LinearAcceleration.vi"("NavX Info In"=w78) -> ("LinearAcceleration"=→"LinearAcceleration":T5, "NavX Info Out"=w82:T4)  [unwired: 9 in]
        n169 = call <vilib>:"Displacement.vi"("NavX Info In"=w78) -> ("Displacement"=→"Displacement":T6, "NavX Info Out"=w80:T4)  [unwired: 9 in]
        n170 = Unbundle By Name(w75) -> ("Yaw"=→"Yaw":dbl)
        n171 = call "FGV Stop.vi"("Init/Read/Write State"=States_for_Action_Engine."Read") -> ("Output node"=w87:bool)  [unwired: 2 in, 1 out]
        n172 = Wait Until Next ms Multiple(millisecond multiple=u32 10) -> ()  [unwired: 1 out]
      }
      n173 = while {
        stop <- w67 stop-if-true
        # "Blackhawk interfacing"
        n174 = call <vilib>:"Blackhawk i2c Open.vi"("I2C Channel"=I2C_Channel."B") -> ("I2C Ref Out"=w73:T17, "error out"=w72:errorcluster)  [unwired: 2 in]
        n175 = call <vilib>:"Blackhawk DIO Read.vi"("I2C Ref In"=w73, "PIN"=u8 0, "error in (no error)"=w72) -> ("I2C Ref Out"=w65:T17, "Value Read"=→"Value Read":bool, "error out"=w66:errorcluster)  [unwired: 3 in]
        n176 = call <vilib>:"Blackhawk Relay.vi"("error in (no error)"=w66, "On/Off"="On/Off", "Relay"=enum8{"Relay 0", "Relay 1", "Relay 2"}."Relay 0", "I2C Ref In"=w65) -> ("error out"=w61:errorcluster, "I2C Ref Out"=w62:T17)  [unwired: 6 in]
        n177 = call <vilib>:"Blackhawk Servo.vi"("error in (no error)"=w61, "Servo Select"=enum16{"Servo 5", "Servo 6"}."Servo 5", "Servo Angle"="Servo Angle", "I2C Ref In"=w62) -> ("error out"=→"Blackhawk error":errorcluster)  [unwired: 6 in, 1 out]
        n178 = call <vilib>:"Blackhawk Servo.vi"() -> ()  [unwired: 10 in, 2 out]
        n179 = call "FGV Stop.vi"("Init/Read/Write State"=States_for_Action_Engine."Read") -> ("Output node"=w67:bool)  [unwired: 2 in, 1 out]
      }
      n180 = while {
        shift-right: [w96] -> _
        shift-left: _ -> [w97]
        stop <- w102 stop-if-true
        w107 = T18 [enum."B/AI0"] items=["Not Connected", "AudioIn/Left", "AudioIn/Right", "C/AI0", "C/AI1", "A/AI0", "A/AI1", "A/AI2", "A/AI3", "A/AI4", "A/AI5", "A/AI6", "A/AI7", "B/AI0", "B/AI1", "B/AI2", "B/AI3", "B/AI4", "B/AI5", "B/AI6", "B/AI7", "AI/AI0", "AI/AI1", "AI/AI2", "AI/AI3", "A/AI0 (DIFF)", "A/AI1 (DIFF)", "A/AI2 (DIFF)", "A/AI3 (DIFF)", "B/AI0 (DIFF)", "B/AI1 (DIFF)", "B/AI2 (DIFF)", "B/AI3 (DIFF)"] ("AI Channel")
        w108 = T18 [enum."A/AI0"] items=["Not Connected", "AudioIn/Left", "AudioIn/Right", "C/AI0", "C/AI1", "A/AI0", "A/AI1", "A/AI2", "A/AI3", "A/AI4", "A/AI5", "A/AI6", "A/AI7", "B/AI0", "B/AI1", "B/AI2", "B/AI3", "B/AI4", "B/AI5", "B/AI6", "B/AI7", "AI/AI0", "AI/AI1", "AI/AI2", "AI/AI3", "A/AI0 (DIFF)", "A/AI1 (DIFF)", "A/AI2 (DIFF)", "A/AI3 (DIFF)", "B/AI0 (DIFF)", "B/AI1 (DIFF)", "B/AI2 (DIFF)", "B/AI3 (DIFF)"] ("AI Channel")
        # "IR + Ultrasonic Sensor Loop"
        n181 = call <vilib>:"Ping.vi"("Mxp Side"=Mxp_Selection."MXP B") -> ("CM"=w95:fxp<+,64,16>)  [unwired: 8 in, 2 out]
        "CM" <- w95
        n182 = call <vilib>:"Sharp IR.vi"("AI Channel"=w108) -> ("Sharp IR Distance"=→"Right IR Sensor":dbl)  [unwired: 8 in, 2 out]
        n183 = call <vilib>:"Sharp IR.vi"("AI Channel"=w107) -> ("Sharp IR Distance"=→"Left IR Sensor":dbl)  [unwired: 8 in, 2 out]
        n184 = Greater Or Equal?(x=w95, y=fxp<+,64,16> 299.0) -> (x >= y?=w98:bool)
        n185 = call <vilib>:"Mean PtByPt.vi"("x"=w95, "sample length"=100) -> ()  [unwired: 2 in, 2 out]
        n186 = Select(t=w97, s=w98, f=w95) -> (s? t:f=w96:fxp<+,64,16>)
        "Ultrasonic sensor" <- w96
        n187 = call "FGV Stop.vi"("Init/Read/Write State"=States_for_Action_Engine."Read") -> ("Output node"=w102:bool)  [unwired: 2 in, 1 out]
        n188 = In Range and Coerce(upper limit=fxp<+,64,16> 250.0, x=w95, lower limit=fxp<+,64,16> 0.0 ("CM")) -> ()  [unwired: 2 out]
        n189 = Wait Until Next ms Multiple(millisecond multiple=u32 10) -> ()  [unwired: 1 out]
      }
      n190 = call <vilib>:"DIO Open.vi"("DIO Channel"=DIO_Channel."C/DIO0") -> ("DIO Info Out"=w2:T20)  [unwired: 9 in, 1 out]
      n191 = while {
        tunnel: w2 -> [w48]
        stop <- w51 stop-if-true
        n192 = Wait (ms)(milliseconds to wait=u32 10) -> ()  [unwired: 1 out]
        n193 = call "FGV Stop.vi"("Init/Read/Write State"=States_for_Action_Engine."Read") -> ("Output node"=w51:bool)  [unwired: 2 in, 1 out]
        n194 = call "Vision Acquisition"("Stop (F)"=w51) -> ("Image Out"=w50:T1, "Stopped"=w47:bool, "error out"=w46:errorcluster)  [unwired: 24 in]
        n195 = Not(x=w47) -> (.not. x?=w43:bool)
        n196 = feedback #1() -> (w41:bool)  [unwired: 1 in]
        n197 = Exclusive Or(1:w41, 2:w43) -> (0:w42:bool)
        n198 = feedback-in #1(w42) -> ()
        n199 = case shown="False" "Camera playback" {
          tunnel: w50 -> [_ w57]
          tunnel: w46 -> [w53 w56]
          tunnel: [_ w55] -> w45
          tunnel: [w53 w54] -> w44
          frame False {
          }
          frame True {
            n200 = call "Red ball detection subVI.vi"("error in"=w56, "Image In"=w57) -> ("error out"=w54:errorcluster, "Image overlay"=w55:T1)
          }
        }
        "Image Out" <- w45
        "Image Processing error" <- w44
        n201 = call <vilib>:"DIO Write.vi"("Input"=w41, "DIO Info In"=w48) -> ()  [unwired: 8 in, 2 out]
      }
      n202 = call <vilib>:"NavX Close.vi"("NavX Info In"=w5) -> ()  [unwired: 10 in, 1 out]
      n203 = call <vilib>:"NavX Close.vi"("NavX Info In"=w9) -> ()  [unwired: 10 in, 1 out]
      n204 = call <vilib>:"NavX Close.vi"("NavX Info In"=w8) -> ()  [unwired: 10 in, 1 out]
      n205 = call <vilib>:"NavX Close.vi"("NavX Info In"=w7) -> ()  [unwired: 10 in, 1 out]
      n206 = call <vilib>:"NavX Close.vi"("NavX Info In"=w6) -> ()  [unwired: 10 in, 1 out]
      n207 = Merge Errors "Merge Errors"(w33, w32) -> (w12:errorcluster)
      n208 = Merge Errors(w18, w12) -> (w14:errorcluster)
      n209 = Destroy User Event(user event=w36, error in=w14) -> ()  [unwired: 1 out]
      n210 = Destroy User Event(user event=w37, error in=w14) -> ()  [unwired: 1 out]
      n211 = Unregister For Events(event registration refnum=w28, error in=w14) -> ()  [unwired: 1 out]
      n212 = Release Queue(queue=w27, error in (no error)=w14) -> ()  [unwired: 1 in, 3 out]
      n213 = Release Queue(queue=w13, error in (no error)=w14) -> ()  [unwired: 1 in, 3 out]
    }
    frame #2 {
    }
  }
